vi "Initialize.vi"(8 "error in (no error)":errorcluster, 11 "Device Item Ref in":T1 format="%.0x") -> (0 "error out":errorcluster, 3 "Device Item Ref out":T1 format="%.0x")   [LabVIEW 2020, in "Communication Bus Template System Explorer.lvlib" / "Implementation.lvlib"]
uses:
  Implementation.lvlib
  <vilib>/NI VeriStand/Custom Device API/Custom Device Item Ref.ctl
  Scripting/Communication Bus Template Scripting.lvlib
  <vilib>/NI VeriStand/Custom Device API/Custom Device API.lvlib
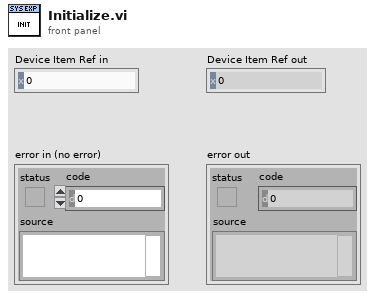
[diagram p1: front panel]
types:
  T1 = typedef "Custom Device API.lvlib/Custom Device Item Ref.ctl" = u64
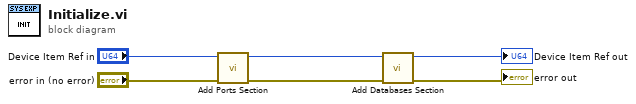
[diagram p0: block diagram]
diagram:
  n1 = call "Add Ports Section.vi"("error in"="error in (no error)", "Custom device Ref"="Device Item Ref in") -> ("error out"=w1:errorcluster, "Custom device Ref out"=w2:T1)  [unwired: 8 in]
  n2 = call "Add Databases Section.vi"("error in"=w1, "Custom device Ref"=w2) -> ("error out"=→"error out":errorcluster, "Custom device Ref out"=→"Device Item Ref out":T1)  [unwired: 8 in]
